vi "ParseUpDefs.vi"(10 "search":string, 11 "Rows":string[](array[string])) -> (0 "left":string, 2 "Names":string[](array[string]), 5 "code":string[](array[string]))   [LabVIEW 2016]
panel:
  out "positions":cluster{i32, i32}[](array[cluster])
  out "def lines":i32[](array[numeric])
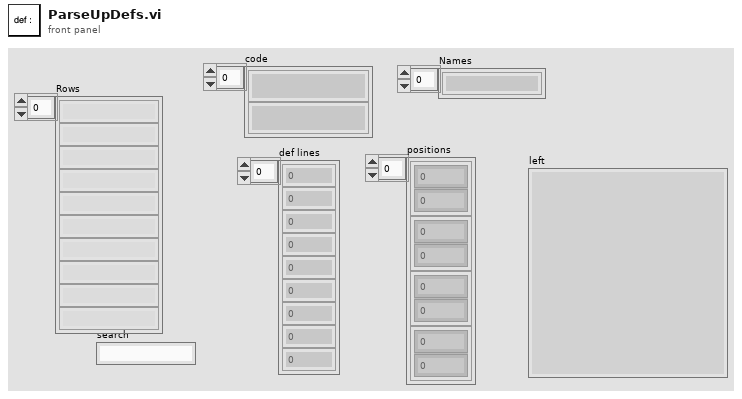
[diagram p1: front panel]
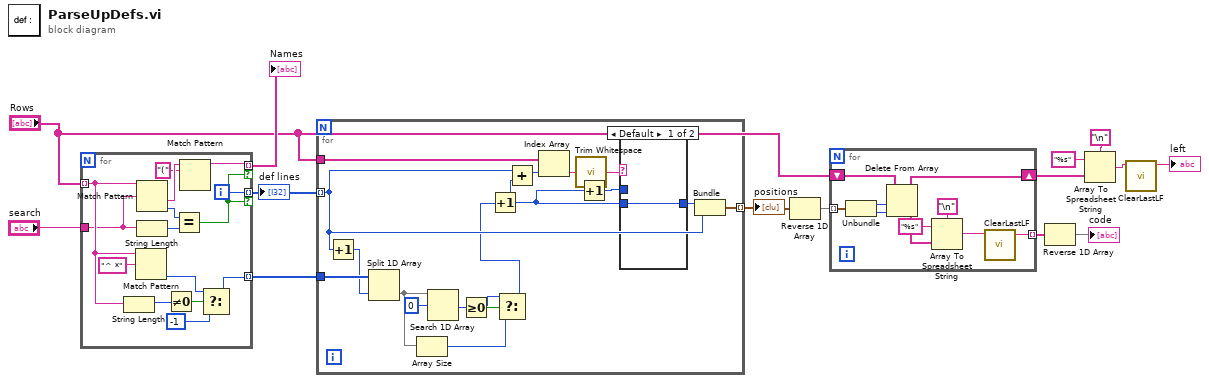
[diagram p0: block diagram]
diagram:
  n1 = for {
    tunnel: "Rows" -> [w21] mode=indexing
    tunnel: [w16] -> w4 mode=indexing
    tunnel: [w26] -> w3 mode=indexing if=w22
    tunnel: [w23] -> w13 mode=indexing if=w22
    tunnel: "search" -> [w15]
    i -> [w26]
    n2 = String Length(string=w21) -> (length=w20:i32)
    n3 = Match Pattern(string=w21, regular expression="^ *") -> (offset past match=w18:i32)  [unwired: 1 in, 3 out]
    n4 = Match Pattern(string=w21, regular expression=w15) -> (after substring=w25:string, offset past match=w28:i32)  [unwired: 1 in, 2 out]
    n5 = String Length(string=w15) -> (length=w27:i32)
    n6 = Not Equal To 0?(x=w20) -> (x != 0?=w19:bool)
    n7 = Equal?(x=w28, y=w27) -> (x = y?=w22:bool)
    n8 = Match Pattern(string=w25, regular expression="(") -> (before substring=w23:string)  [unwired: 1 in, 3 out]
    n9 = Select(t=w18, s=w19, f=-1) -> (s? t:f=w16:i32)
  }
  "def lines" <- w3
  "Names" <- w13
  n10 = for {
    tunnel: w3 -> [w38] mode=indexing
    tunnel: w4 -> [w46]
    tunnel: [w44] -> w5 mode=indexing
    tunnel: "Rows" -> [w42]
    n11 = Increment(x=w38) -> (x+1=w43:i32)
    n12 = Split 1D Array(array=w46, index=w43) -> (second subarray=w32:i32[])  [unwired: 1 out]
    n13 = Array Size(array=w32) -> (size(s)=w30:i32)
    n14 = Search 1D Array(1D array=w32, element=0) -> (index of element=w33:i32)  [unwired: 1 in]
    n15 = Greater Or Equal To 0?(x=w33) -> (x >= 0?=w34:bool)
    n16 = Select(t=w33, s=w34, f=w30) -> (s? t:f=w31:i32)
    n17 = Increment(x=w31) -> (x+1=w35:i32)
    n18 = Add(x=w38, y=w35) -> (x+y=w37:i32)
    n19 = Index Array(array=w42, index=w37) -> (element=w41:string)
    n20 = call <vilib>:"Trim Whitespace.vi"("string"=w41) -> ("trimmed string"=w39:string)  [unwired: 1 in]
    n21 = Increment(x=w35) -> (x+1=w36:i32)
    n22 = case shown="Default" w39 {
      tunnel: [w47 w48] -> w40
      tunnel: w35 -> [w47 _]
      tunnel: w36 -> [_ w48]
      frame Default {
      }
      frame "" {
      }
    }
    n23 = Bundle(w40, w38) -> (w44:cluster{i32, i32})  [unwired: 1 in]
  }
  "positions" <- w5
  n24 = Reverse 1D Array(array=w5) -> (reversed array=w6:cluster{i32, i32}[])
  n25 = for {
    tunnel: w6 -> [w58] mode=indexing
    shift-right: [w54] -> w10
    shift-left: "Rows" -> [w57]
    tunnel: [w49] -> w7 mode=indexing
    n26 = Unbundle(w58) -> (w56:i32, w55:i32)
    n27 = Delete From Array(array=w57, length=w56, index=w55) -> (deleted portion=w53:string[], array with subset deleted=w54:string[])
    n28 = Array To Spreadsheet String(delimiter (Tab)="\n", array=w53, 3:"%s" ("format string")) -> (spreadsheet string=w50:string)
    n29 = call "ClearLastLF.vi"("spreadsheet string in"=w50) -> ("spreadsheet string out"=w49:string)  [unwired: 10 in]
  }
  n30 = Reverse 1D Array(array=w7) -> (reversed array=→"code":string[])
  n31 = Array To Spreadsheet String(delimiter (Tab)="\n", array=w10, 3:"%s" ("format string")) -> (spreadsheet string=w1:string)
  n32 = call "ClearLastLF.vi"("spreadsheet string in"=w1) -> ("spreadsheet string out"=→"left":string)  [unwired: 10 in]
